vi "globalvariables.vi"() -> ()   [LabVIEW 2014]
panel:
  in  "Numeric":i8=-1
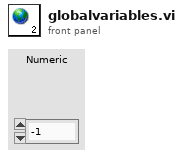
[diagram p1: front panel]
diagram:
